vi "LVClass_ComputePhaseSet ctor from TypePhase.vi"(0 "ComputePhaseSet in":refnum<class "ComputePhaseSet.lvclass">, 5 "TypePhase":T1, 11 "error in (no error)":errorcluster) -> (4 "ComputePhaseSet out":refnum<class "ComputePhaseSet.lvclass">, 15 "error out":errorcluster)   [LabVIEW 2020, in "ComputePhaseSet.lvclass"]
doc: "ComputePhaseSet constructor from TypePhase value.\n\n--------------------------------------------------------------------------------\n\n<B>ComputePhaseSetIn </B> : Constant Pointer to ComputePhaseSet object.\n<B>ComputePhaseSetOut </B> : Constant Pointer to ComputePhaseSet object.\n<B>TypePhase </B> : TypePhase Polynomial bases enumeration.\n<B>ErrorIn </B> : Error\n<B>ErrorOut </B> : Error\n\n--------------------------------------------------------------------------------"
uses:
  ComputePhaseSet.lvclass
  WavefrontReconstructionMode.ctl
  Handle creation.ctl
  ComputePhaseSet.lvclass/ComputePhaseSet.ctl
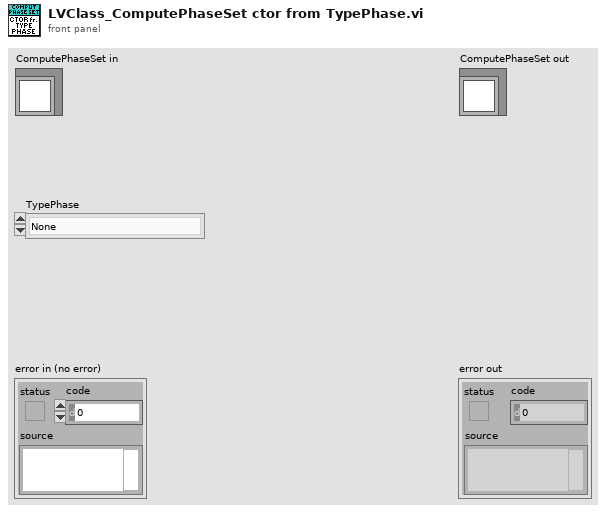
[diagram p1: front panel]
types:
  T1 = typedef "WavefrontReconstructionMode.ctl" = enum16{"None", "Modal_Legendre", "Modal_Zernike", "Zonal", "Modal_Zonal_Zernike", "Modal_Zonal_Legendre"}
  T2 = typedef "Handle creation.ctl" = enum16{"By ctor", "By write function"}
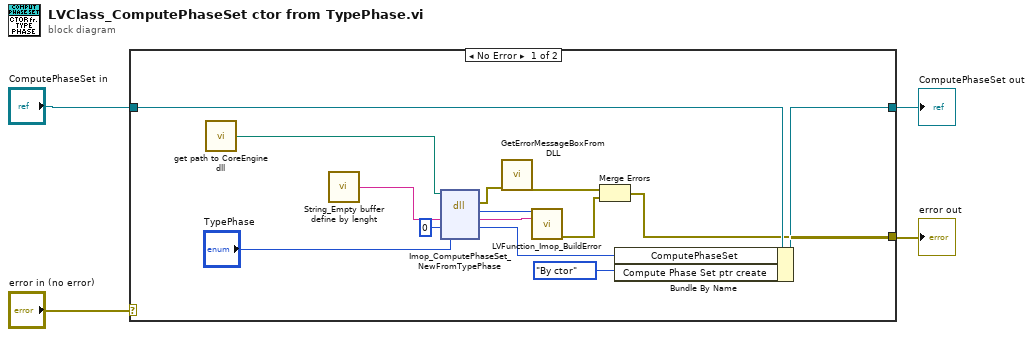
[diagram p0: block diagram]
diagram:
  n1 = case shown="No Error" "error in (no error)" {
    selector: "error in (no error)" -> [_ w20]
    tunnel: [w5 w20] -> w1
    tunnel: [w12 w19] -> w3
    tunnel: "ComputePhaseSet in" -> [w13 w19]
    frame No Error {
      n2 = call "get path to CoreEngine dll.vi"() -> ("path to c_interface_vc100.dll"=w10:path)  [unwired: 12 in, 3 out]
      n3 = call "String_Empty buffer define by lenght.vi"() -> ("Empty buffer"=w11:string)  [unwired: 1 in]
      n4 = dll-call lib="D:/soft/HASO_v3/SVN_trunk/ImOpCoreEngine4_LV2011/DLLs/c_interface_vc100.dll" fn="Imop_ComputePhaseSet_NewFromTypePhase"(path in=w10, "message"=w11, "objet"=0, "TypePhase"="TypePhase") -> (error out=w9:errorcluster, "return type"=w16:i32, "message"=w15:string, "objet"=w14:i32)  [unwired: 3 in, 1 out]
      n5 = call "GetErrorMessageBoxFromDLL.vi"("error IN"=w9) -> ("error OUT"=w7:errorcluster)  [unwired: 10 in]
      n6 = call "LVFunction_Imop_BuildError.vi"("code"=w16, "String to Prepend to source (\"\")"=w15) -> ("error out"=w6:errorcluster)  [unwired: 13 in]
      n7 = Merge Errors(w7, w6) -> (w5:errorcluster)
      n8 = Bundle By Name(cluster=w13, "ComputePhaseSet"=w14, "Compute Phase Set ptr create"=Handle_creation."By ctor" ("Haso ptr create")) -> (w12:refnum<class "ComputePhaseSet.lvclass">)
    }
    frame Error {
    }
  }
  "error out" <- w1
  "ComputePhaseSet out" <- w3
